vi "testTcpServerTel.vi"(8 "error in (no error)":errorcluster) -> (0 "error out":errorcluster)   [LabVIEW 2018]
doc: "Test TcpServerTel class."
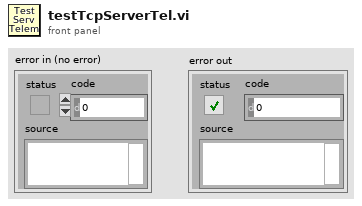
[diagram p1: front panel]
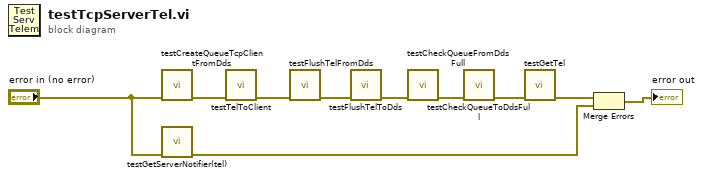
[diagram p0: block diagram]
diagram:
  n1 = call "testCreateQueueTcpClientFromDds.vi"("error in (no error)"="error in (no error)") -> ("error out"=w10:errorcluster)  [unwired: 10 in]
  n2 = call "testGetServerNotifier(tel).vi"("error in (no error)"="error in (no error)") -> ("error out"=w1:errorcluster)  [unwired: 10 in]
  n3 = call "testTelToClient.vi"("error in (no error)"=w10) -> ("error out"=w9:errorcluster)  [unwired: 10 in]
  n4 = call "testFlushTelFromDds.vi"("error in (no error)"=w9) -> ("error out"=w8:errorcluster)  [unwired: 10 in]
  n5 = call "testFlushTelToDds.vi"("error in (no error)"=w8) -> ("error out"=w5:errorcluster)  [unwired: 10 in]
  n6 = call "testCheckQueueFromDdsFull.vi"("error in (no error)"=w5) -> ("error out"=w7:errorcluster)  [unwired: 10 in]
  n7 = call "testCheckQueueToDdsFull.vi"("error in (no error)"=w7) -> ("error out"=w4:errorcluster)  [unwired: 10 in]
  n8 = call "testGetTel.vi"("error in (no error)"=w4) -> ("error out"=w6:errorcluster)  [unwired: 10 in]
  n9 = Merge Errors(w6, w1) -> (→"error out":errorcluster)
